vi "String slicer.vi"(0 "Multiline String":string) -> (1 "Array of numbers with spaces":string[](array[string]), 2 "Array of variable names":string[](array[string]))   [LabVIEW 2013]
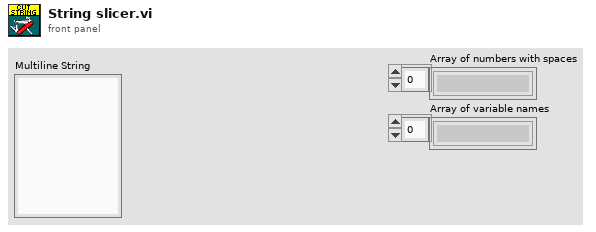
[diagram p1: front panel]
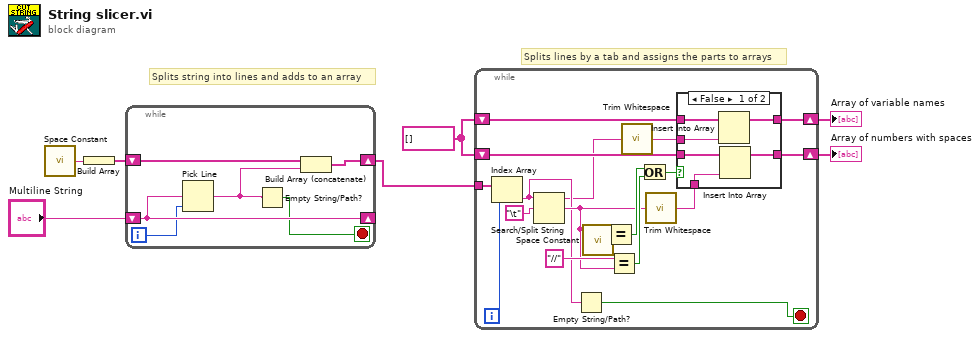
[diagram p0: block diagram]
diagram:
  w2 = string[] []
  # "Splits lines by a tab and assigns the parts to arrays"
  # "Splits string into lines and adds to an array"
  n1 = call <vilib>:"Space Constant.vi"() -> ("String"=w4:string)
  n2 = Build Array(w4) -> (w6:string[])
  n3 = while {
    shift-right: [w13] -> w5
    shift-left: w6 -> [w12]
    shift-right: [w11] -> _
    shift-left: "Multiline String" -> [w11]
    i -> [w10]
    stop <- w8 stop-if-true
    n4 = Pick Line(multi-line string=w11, line index=w10) -> (output string=w9:string)  [unwired: 1 in]
    n5 = Empty String/Path?(string/path=w9) -> (empty?=w8:bool)
    n6 = Build Array (concatenate)(w12, w9) -> (w13:string[])
  }
  n7 = while {
    shift-right: [w31] -> w3
    shift-left: w2 -> [w30]
    tunnel: w5 -> [w28]
    shift-right: [w20] -> w1
    shift-left: w2 -> [w19]
    i -> [w27]
    stop <- w29 stop-if-true
    n8 = Index Array(array=w28, index=w27) -> (element=w16:string)
    n9 = Search/Split String(string=w16, search string/char (-)="\t") -> (substring before match=w14:string, match + rest of string=w17:string)  [unwired: 1 in, 1 out]
    n10 = Empty String/Path?(string/path=w16) -> (empty?=w29:bool)
    n11 = call <vilib>:"Space Constant.vi"() -> ("String"=w23:string)
    n12 = Equal?(x=w17, y=w23) -> (x = y?=w25:bool)
    n13 = Equal?(x="//", y=w17) -> (x = y?=w24:bool)
    n14 = call <vilib>:"Trim Whitespace.vi"("string"=w14) -> ("trimmed string"=w15:string)  [unwired: 1 in]
    n15 = Or(x=w25, y=w24) -> (x .or. y?=w26:bool)
    n16 = call <vilib>:"Trim Whitespace.vi"("string"=w17) -> ("trimmed string"=w18:string)  [unwired: 1 in]
    n17 = case shown="False" w26 {
      tunnel: [w37 w39] -> w31
      tunnel: w30 -> [w36 w39]
      tunnel: w18 -> [w35 _]
      tunnel: [w34 w38] -> w20
      tunnel: w19 -> [w33 w38]
      tunnel: w15 -> [w32 _]
      frame False {
        n18 = Insert Into Array(array=w33, new element=w32) -> (w34:string[])  [unwired: 1 in]
        n19 = Insert Into Array(array=w36, new element=w35) -> (w37:string[])  [unwired: 1 in]
      }
      frame True {
      }
    }
  }
  "Array of numbers with spaces" <- w3
  "Array of variable names" <- w1
